vi "Call vi .vi"(8 "error in (no error)":errorcluster, 11 "DAQCascade512II":refnum<class "DAQCascade512II.lvclass">) -> (0 "error out":errorcluster, 3 "DAQCascade512II 2":refnum<class "DAQCascade512II.lvclass">)   [LabVIEW 2012]
uses:
  DAQCascade512II.lvclass
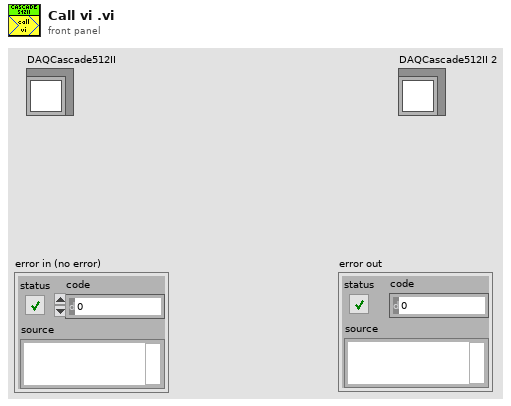
[diagram p1: front panel]
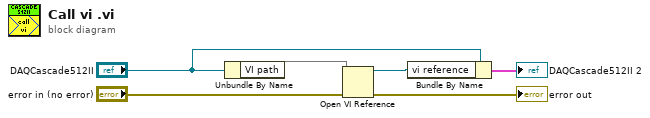
[diagram p0: block diagram]
diagram:
  n1 = Unbundle By Name("DAQCascade512II") -> ("VI path"=w6)
  n2 = Open VI Reference(vi path=w6, error in (no error)="error in (no error)") -> (vi reference=w5:refnum<vi>, error out=→"error out":errorcluster)  [unwired: 4 in]
  n3 = Bundle By Name(cluster="DAQCascade512II", "vi reference"=w5) -> (→"DAQCascade512II 2":cluster{})
